vi "Write Payload Mask.vi"(8 "error in":errorcluster, 10 "Cases to Skip Payload":u8[](array[numeric]), 11 "OOB in":refnum<class "CIFOutOfBand.lvclass">) -> (0 "error out":errorcluster, 3 "OOB out":refnum<class "CIFOutOfBand.lvclass">)   [LabVIEW 2021, in "CIFOutOfBand.lvclass"]
uses:
  CIFOutOfBand.lvclass
  CIFOutOfBand.lvclass/CIFOutOfBand.ctl
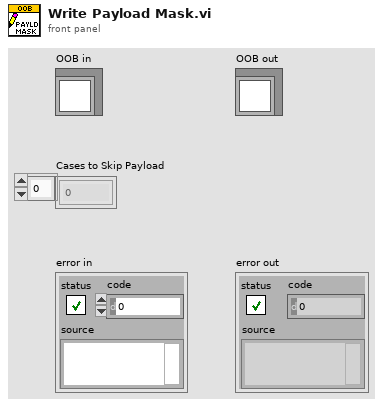
[diagram p1: front panel]
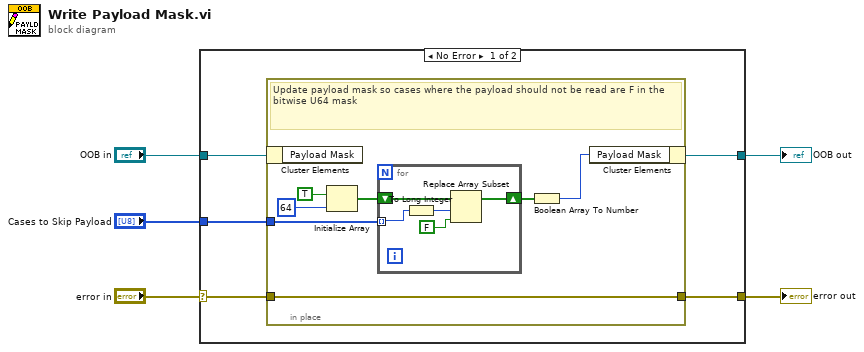
[diagram p0: block diagram]
diagram:
  n1 = case shown="No Error" "error in" {
    selector: "error in" -> [w8 w24]
    tunnel: [w7 w24] -> w5
    tunnel: [w9 w23] -> w4
    tunnel: "OOB in" -> [w10 w23]
    tunnel: "Cases to Skip Payload" -> [w6 _]
    frame No Error {
      n2 = in-place {
        in-place-border: w8 -> [w17]
        in-place-border: [w17] -> w7
        in-place-border: w6 -> [w16]
        # "Update payload mask so cases where the payload should not be read are F in the bitwise U64 mask"
        n3 = in-place-cluster #1(w10) -> ()  [unwired: 1 out]
        n4 = Initialize Array(TRUE, 64 ("dimension size")) -> (w13:bool[])
        n5 = for {
          tunnel: w16 -> [w21] mode=indexing
          shift-right: [w18] -> w12
          shift-left: w13 -> [w22]
          n6 = To Long Integer(number=w21) -> (32bit integer=w20:i32)
          n7 = Replace Array Subset(array=w22, new element=FALSE ("new element/subarray"), index=w20) -> (w18:bool[])
        }
        n8 = Boolean Array To Number(Boolean array=w12) -> (number=w11:u64)
        n9 = in-place-cluster #1("Payload Mask"=w11) -> (w9:refnum<class "CIFOutOfBand.lvclass">)
      }
    }
    frame Error {
    }
  }
  "error out" <- w5
  "OOB out" <- w4
